vi "Servo Open.vi"   [LabVIEW 2014, in "LMH-LINX.lvlib" / "Servo.lvlib"]
uses:
  Servo.lvlib
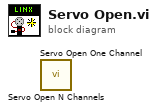
[diagram p0: block diagram]
diagram:
  n1 = call "Servo Open N Channels.vi"() -> ()  [unwired: 10 in, 2 out]
  n2 = call "Servo Open One Channel.vi"() -> ()  [unwired: 10 in, 2 out]
